vi "String2Array.vi"(1 "R_message 1":string) -> (0 "Array 2":string[](array[string]))   [LabVIEW 2021]
panel:
  out "after substring 2":string
  out "before substring 2":string
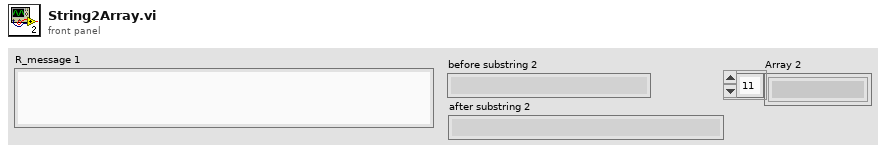
[diagram p1: front panel]
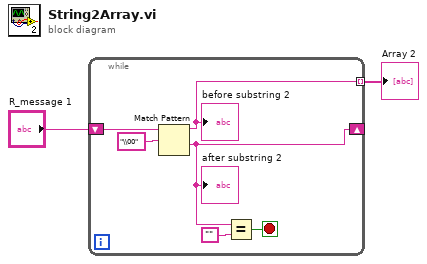
[diagram p0: block diagram]
diagram:
  n1 = while {
    tunnel: [w7] -> w2 mode=indexing
    shift-right: [w3] -> _
    shift-left: "R_message 1" -> [w5]
    stop <- w6 stop-if-true
    n2 = Match Pattern(string=w5, regular expression="\\00") -> (before substring=w7:string, after substring=w3:string)  [unwired: 1 in, 2 out]
    "before substring 2" <- w7
    "after substring 2" <- w3
    n3 = Equal?(x=w3, y="") -> (x = y?=w6:bool)
  }
  "Array 2" <- w2
